vi "single-rev.vi"() -> ()   [LabVIEW 2020]
uses:
  rev_meas/Device_state.ctl
  GlobalDeviceNum1.vi
  support/Message Queue/Message Queue.lvlib
  support/User Event - Stop/User Event - Stop.lvlib
  setup/support/rev_setup.lvlib
  rev_meas/rev_meas.lvlib
  bas_meas/bas_meas.lvlib
panel:
  out "待处理删除数量":i32
  in  "校准":bool
  in  "EM设置":bool
  in  "HW设置":bool
  in  "退出":bool
  in  "开始":bool
  in  "选项卡控件":enum32{"当前结果", "记录结果", "分析结果"}(tab)
  out "当前混响频谱图":cluster{dbl[], "所有X坐标":dbl[]}(graph)
  in  "T1":bool
  in  "T2":bool
  in  "当前混响结果":i32(listbox)
  out "测量状态":string
  out "队列中元素数量":i32
  in  "deletelineT1":bool
  in  "clearlistT1":bool
  in  "deletelineT2":bool
  in  "clearlistT2":bool
  in  "T1结果":i32(listbox)
  in  "T2结果":i32(listbox)
  in  "All results":i32(listbox)
  in  "analysis":bool
  out "欢迎":string="欢迎使用"
  out "日期/时间字符串":string
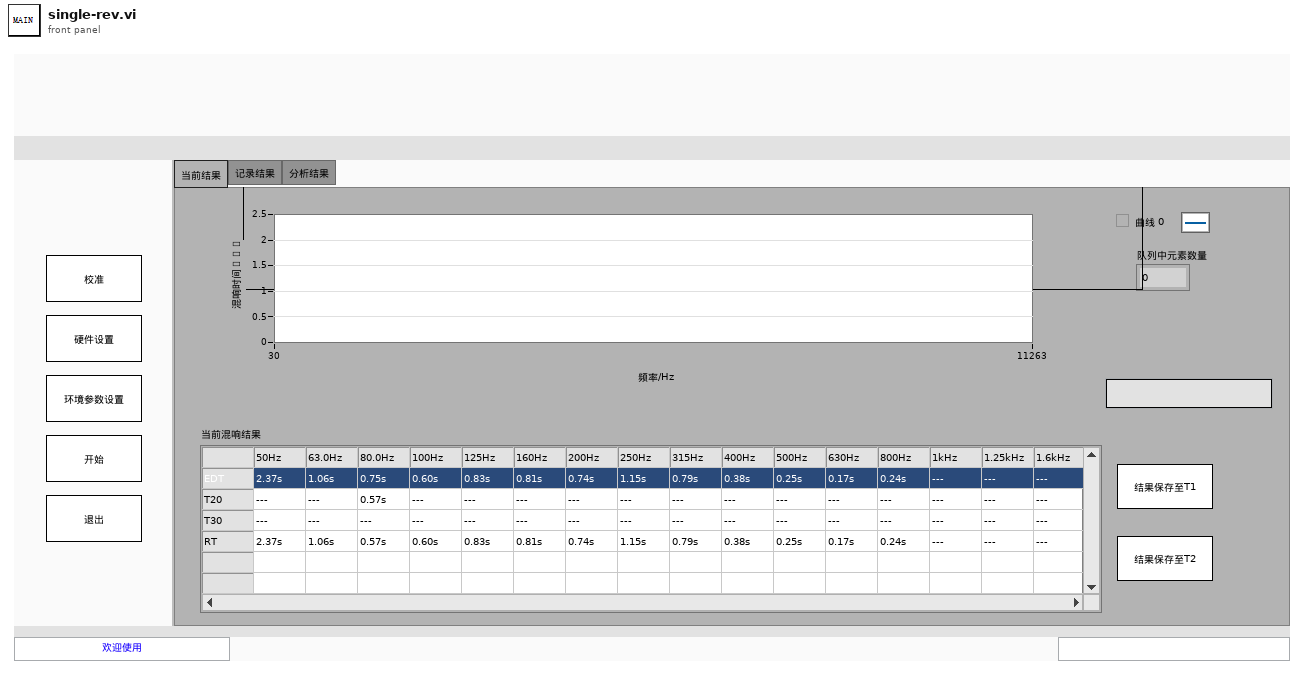
[diagram p1: front panel]
types:
  T1 = typedef "rev_meas.lvlib/Device_state.ctl" = enum16{"Idel", "testing", "stoped"}
  T2 = typedef "Message Queue.lvlib/All Message Queues.ctl" = cluster{"UI":refnum<queue>, "采集":refnum<queue>, "记录":refnum<queue>}
  T3 = cluster{"T1":dbl[], "T2":dbl[], "A1":dbl[], "A2":dbl[], "AT":dbl[], "Aobj":dbl[], "αs":dbl[]}
  T4 = cluster{"T1":string[], "T2":string[], "A1":string[], "A2":string[], "AT":string[], "Aobj":string[], "αs":string[]}
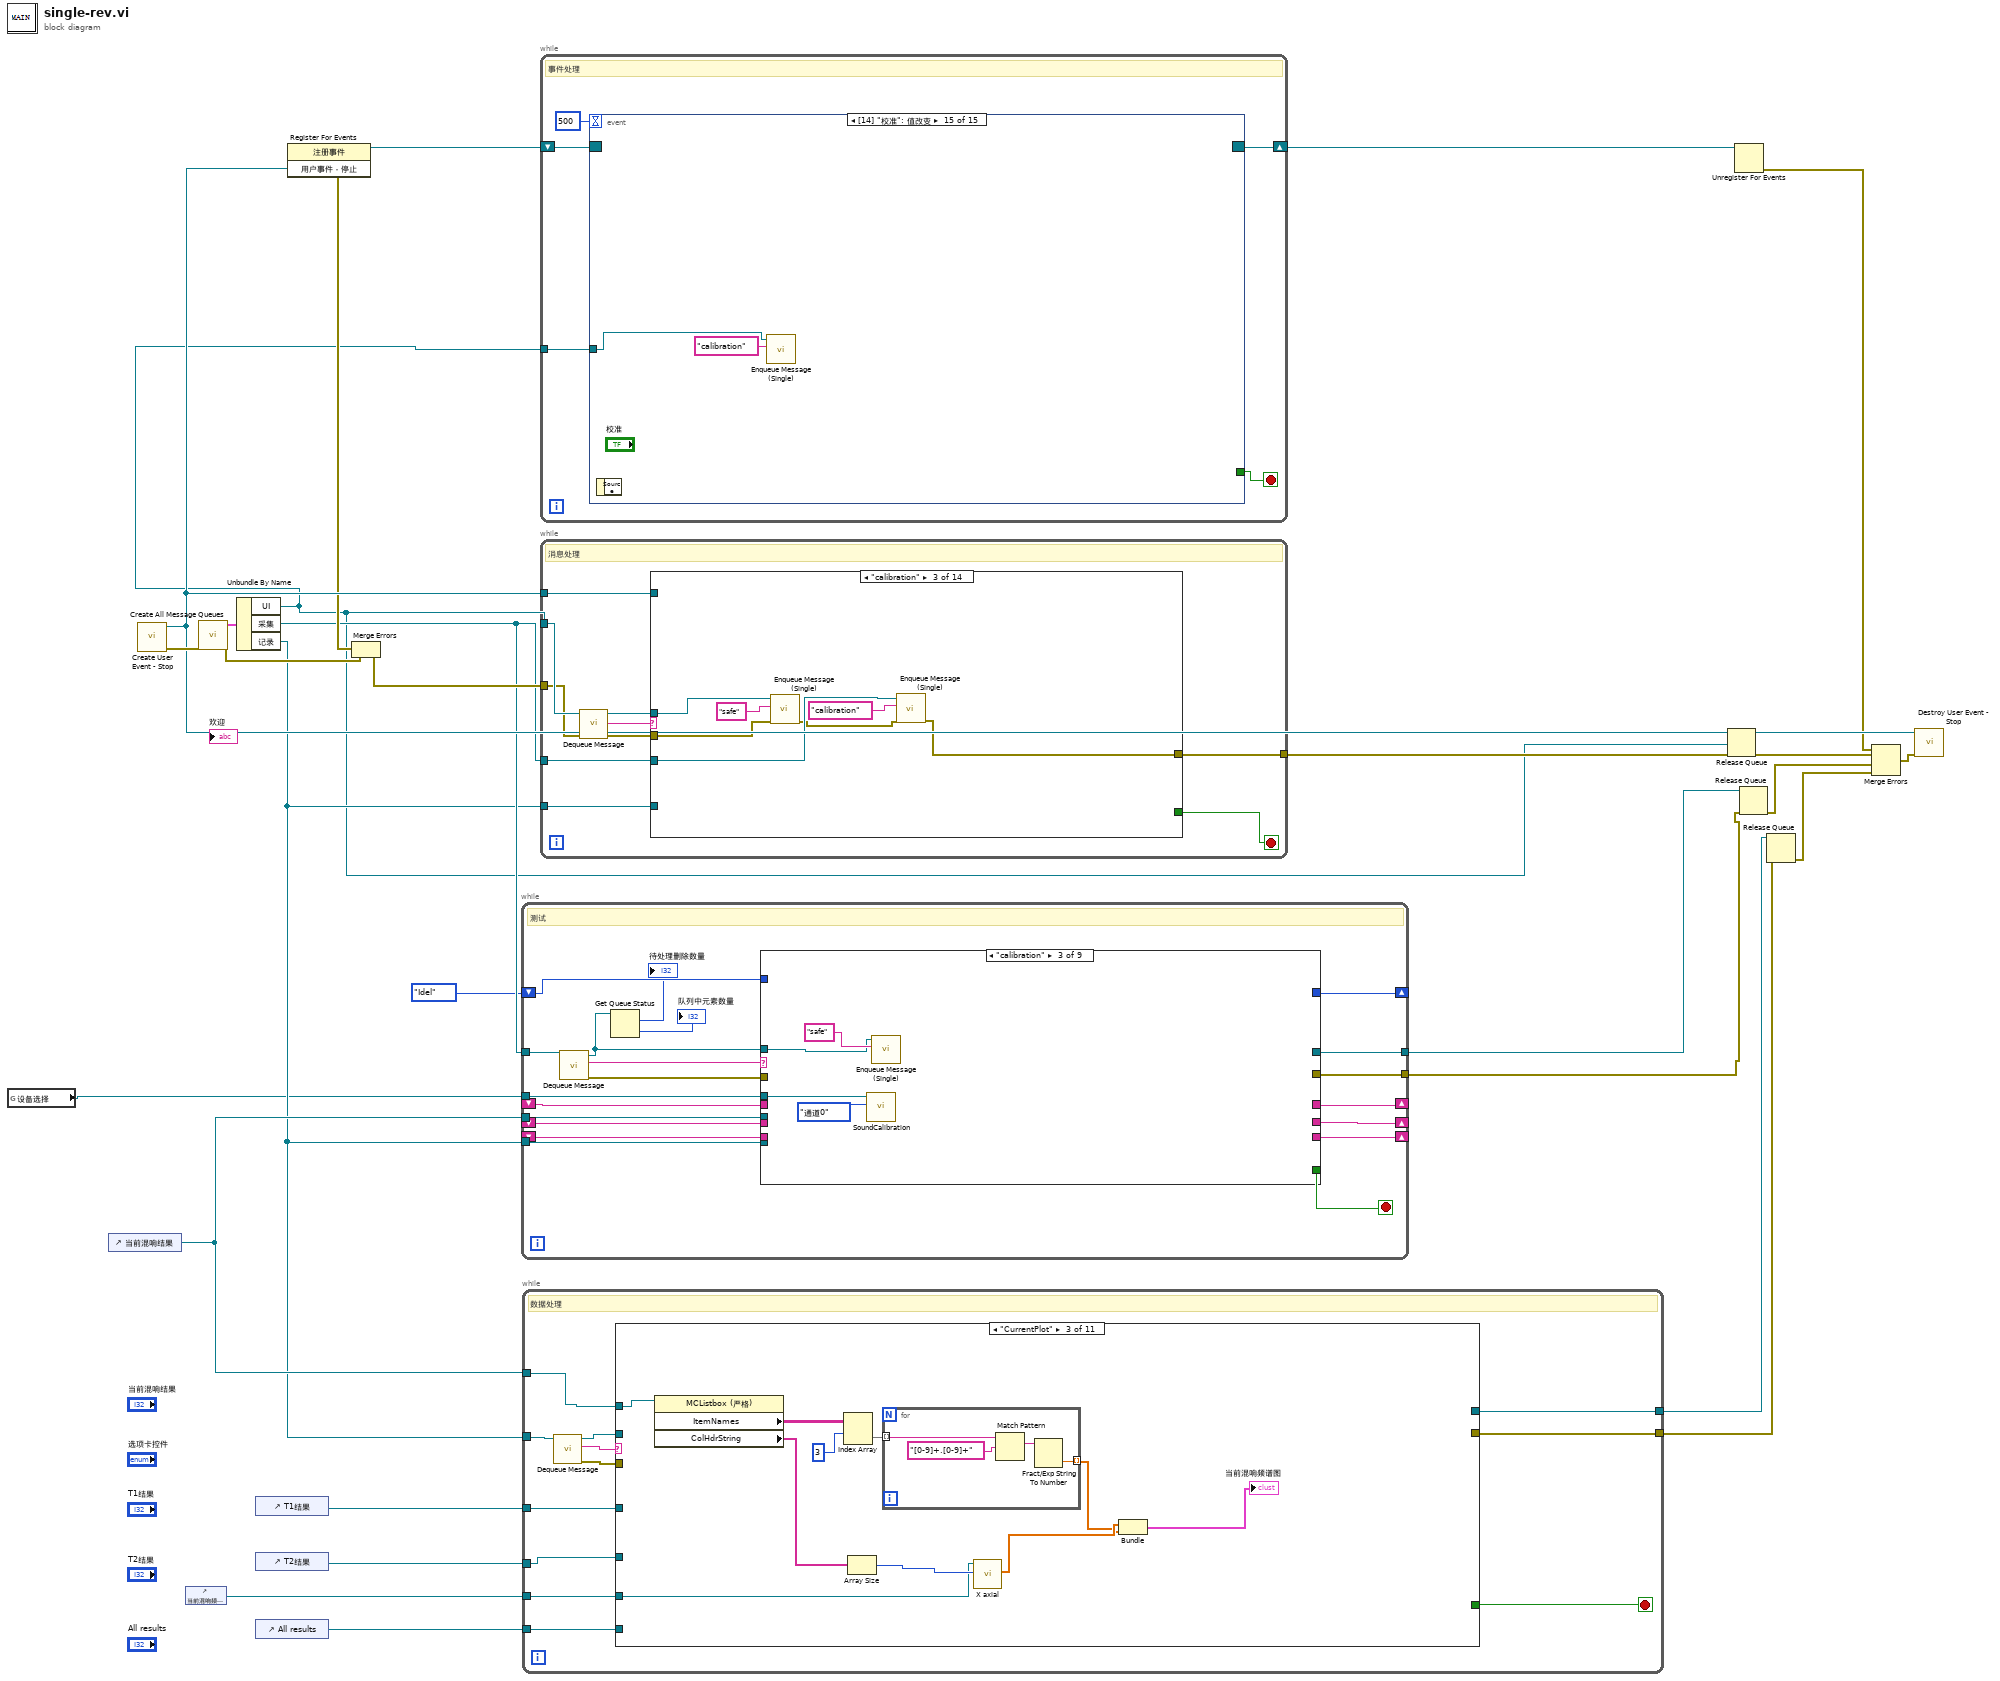
[diagram p0: block diagram]
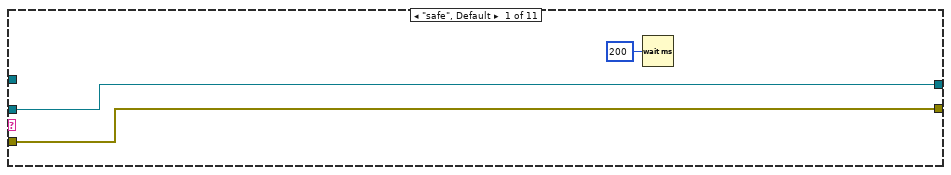
[diagram p2: hidden frame]
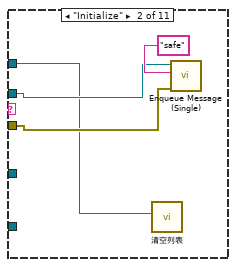
[diagram p3: hidden frame]
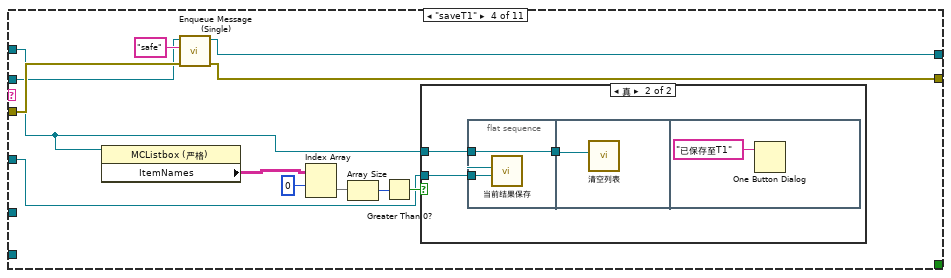
[diagram p4: hidden frame]
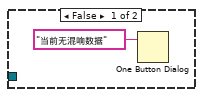
[diagram p5: hidden frame]
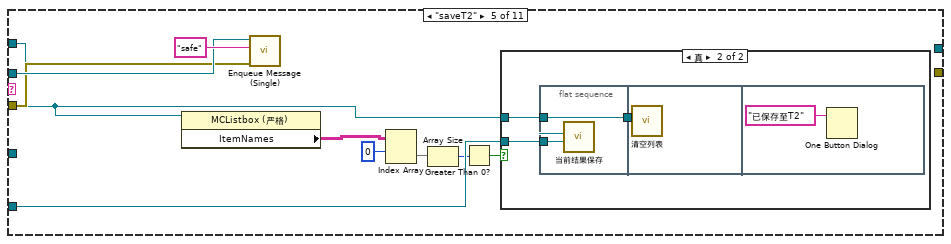
[diagram p6: hidden frame]
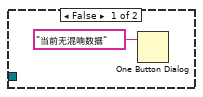
[diagram p7: hidden frame]
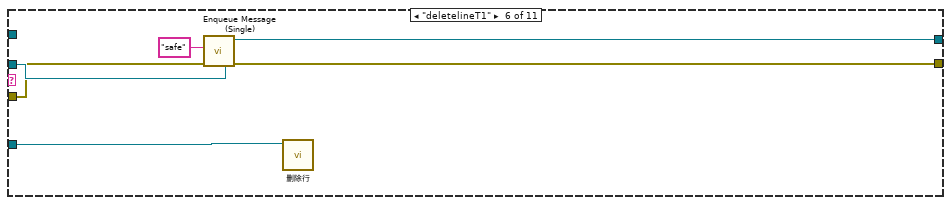
[diagram p8: hidden frame]
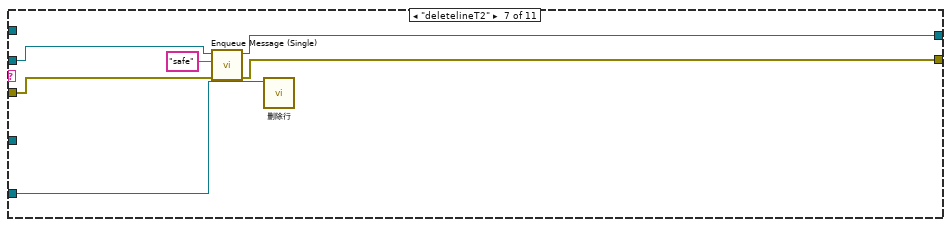
[diagram p9: hidden frame]
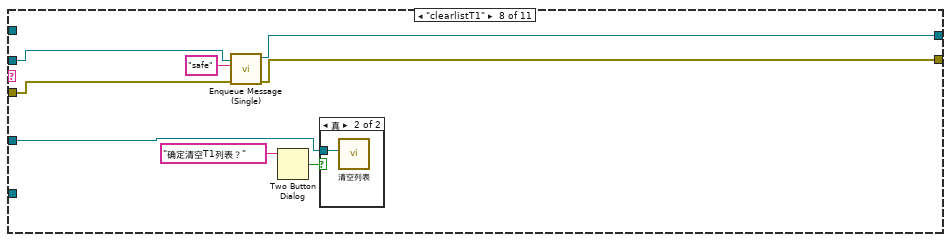
[diagram p10: hidden frame]
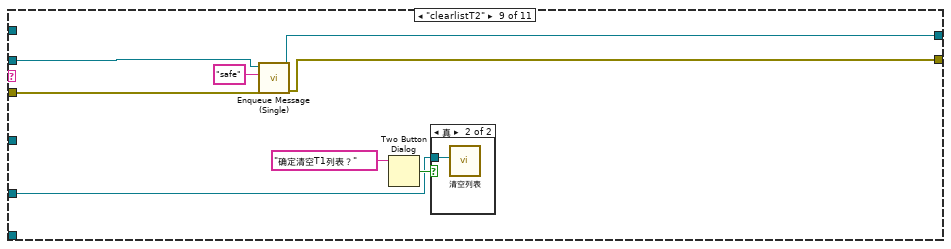
[diagram p12: hidden frame]
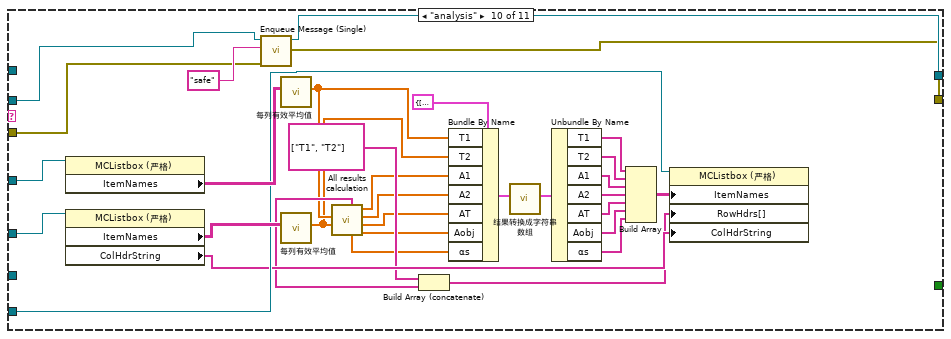
[diagram p14: hidden frame]
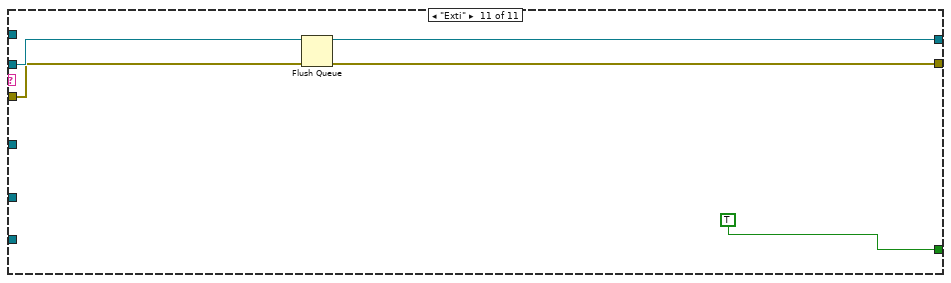
[diagram p15: hidden frame]
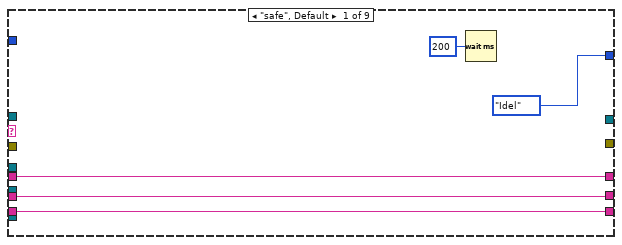
[diagram p16: hidden frame]
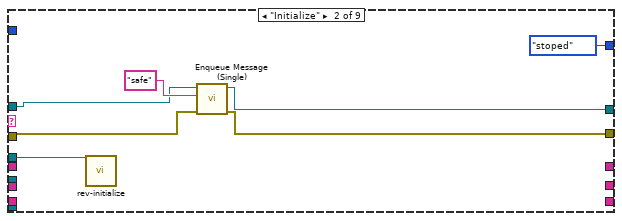
[diagram p17: hidden frame]
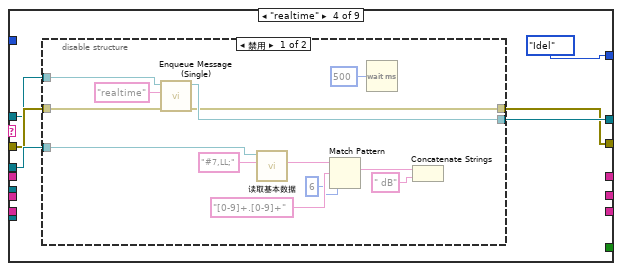
[diagram p18: hidden frame]
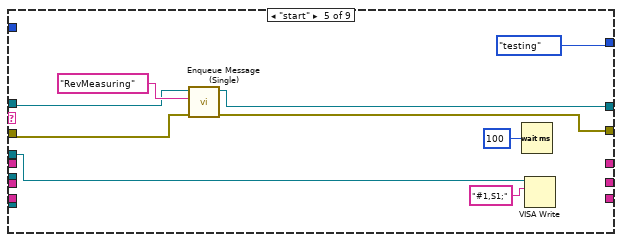
[diagram p20: hidden frame]
diagram:
  n1 = global read "GlobalDeviceNum1.vi" "设备选择"() -> (w4:refnum<visa-resource-name>)
  n2 = control-ref of="当前混响结果"() -> (w9:refnum<vi>)
  n3 = call "Create User Event - Stop.vi"() -> ("error out"=w26:cluster{"状态":bool, "代码":i32, "源":string}, "用户事件－停止"=w25:refnum<user-event>)  [unwired: 10 in]
  n4 = control-ref of="当前混响频谱图"() -> (w2:refnum<vi>)
  n5 = call "Create All Message Queues.vi"("error in (no error)"=w26) -> ("error out"=w23:cluster{"状态":bool, "代码":i32, "源":string}, "消息队列输出"=w28:T2)  [unwired: 9 in]
  n6 = Unbundle By Name(w28) -> ("UI"=w3:refnum<queue>, "采集"=w19:refnum<queue>, "记录"=w6:refnum<queue>)
  n7 = control-ref of="T1结果"() -> (w8:refnum<vi>)
  n8 = control-ref of="T2结果"() -> (w7:refnum<vi>)
  n9 = control-ref of="All results"() -> (w5:refnum<vi>)
  n10 = register-events(w25) -> (reference out=w27:refnum<event-registration>, error out=w22:errorcluster)  [unwired: 2 in]
  n11 = Merge Errors(w22, w23) -> (w21:errorcluster)
  n12 = while {
    tunnel: w4 -> [w46]
    tunnel: w9 -> [w43]
    tunnel: [w41] -> w11
    tunnel: w6 -> [w40]
    shift-right: [w39] -> _
    shift-left: _ -> [w36]
    shift-right: [w38] -> _
    shift-left: _ -> [w35]
    shift-right: [w37] -> _
    shift-left: _ -> [w34]
    shift-right: [w33] -> _
    shift-left: Device_state."Idel" ("枚举") -> [w32]
    tunnel: w19 -> [w48]
    tunnel: [w42] -> w15
    stop <- w44 stop-if-true
    # "测试"
    n13 = call "Dequeue Message.vi"("消息队列"=w48) -> ("error out"=w47:cluster{"状态":bool, "代码":i32, "源":string}, "消息"=w45:string, "消息队列副本"=w30:refnum<queue>)  [unwired: 7 in, 1 out]
    n14 = Get Queue Status(queue=w30) -> (# pending remove=→"待处理删除数量":i32, # elements in queue=→"队列中元素数量":i32)  [unwired: 2 in, 6 out]
    n15 = case shown="\"calibration\"" w45 {
      tunnel: w30 -> [_ w59 w61 w67 w88 w93 w133 w137 w145]
      tunnel: w47 -> [_ w58 _ w68 w87 w100 w132 w136 w143]
      tunnel: w46 -> [_ w55 w64 w69 w90 w102 _ w139 _]
      tunnel: [_ _ _ _ _ _ _ _ TRUE] -> w44
      tunnel: w43 -> [_ _ _ _ _ _ w121 _ _]
      tunnel: [_ w57 _ w66 w86 w95 w118 _ w144] -> w42
      tunnel: [_ w56 _ w65 w85 w94 w113 _ w142] -> w41
      tunnel: w40 -> [_ _ _ _ _ _ w119 _ _]
      tunnel: [w52 _ _ _ _ w99 _ _ _] -> w39
      tunnel: [w51 _ _ _ _ w98 _ _ _] -> w38
      tunnel: [w50 _ _ _ _ w97 _ _ _] -> w37
      tunnel: w36 -> [w52 _ _ _ _ _ w131 _ _]
      tunnel: w35 -> [w51 _ _ _ _ _ w130 _ _]
      tunnel: w34 -> [w50 _ _ _ _ _ w129 _ _]
      tunnel: [Device_state."Idel" ("枚举") Device_state."stoped" ("枚举") _ Device_state."Idel" ("枚举") Device_state."testing" ("枚举") Device_state."testing" ("枚举") Device_state."Idel" ("枚举") _ _] -> w33
      tunnel: w32 -> [_ _ _ _ _ _ _ _ _]
      frame "safe", Default {
        n16 = Wait (ms)(milliseconds to wait=u32 200 ("等待时间（毫秒）")) -> ()  [unwired: 1 out]
      }
      frame "Initialize" {
        n17 = call "rev-initialize.vi"("设备选择"=w55) -> ()  [unwired: 11 in]
        n18 = call "Enqueue Message (Single).vi"("error in (no error)"=w58, "消息"="safe", "消息队列"=w59) -> ("error out"=w56:cluster{"状态":bool, "代码":i32, "源":string}, "消息队列副本"=w57:refnum<queue>)  [unwired: 7 in]
      }
      frame "calibration" {
        n19 = call "SoundCalibration.vi"("通道选择"=enum16{"通道0", "通道1", "通道2", "通道3"}."通道0", "设备选择"=w64) -> ()  [unwired: 10 in]
        n20 = call "Enqueue Message (Single).vi"("消息"="safe", "消息队列"=w61) -> ()  [unwired: 8 in, 2 out]
      }
      frame "realtime" {
        n21 = disable-structure shown="禁用" {
          disable-tunnel: w69 -> [w83 _]
          disable-tunnel: w68 -> [w82 _]
          disable-tunnel: w67 -> [w81 _]
          disable-tunnel: [w80 _] -> w66
          disable-tunnel: [w79 _] -> w65
          frame Disabled {
            n22 = call "Enqueue Message (Single).vi"("error in (no error)"=w82, "消息"="realtime", "消息队列"=w81) -> ("error out"=w79:cluster{"状态":bool, "代码":i32, "源":string}, "消息队列副本"=w80:refnum<queue>)  [unwired: 7 in]
            n23 = call "读取基本数据.vi"("写入缓冲区"="#7,LL;", "设备选择"=w83) -> ("read buffer"=w77:string)  [unwired: 9 in]
            n24 = Match Pattern(string=w77, regular expression="[0-9]+.[0-9]+" ("正则表达式"), offset (0)=6 ("偏移量(0)")) -> (match substring=w78:string)  [unwired: 3 out]
            n25 = Wait (ms)(milliseconds to wait=u32 500 ("等待时间（毫秒）")) -> ()  [unwired: 1 out]
            n26 = Concatenate Strings(w78, " dB" ("字符串")) -> ()  [unwired: 1 out]
          }
          frame Enabled {
          }
        }
      }
      frame "start" {
        n27 = call "Enqueue Message (Single).vi"("error in (no error)"=w87, "消息"="RevMeasuring", "消息队列"=w88) -> ("error out"=w85:cluster{"状态":bool, "代码":i32, "源":string}, "消息队列副本"=w86:refnum<queue>)  [unwired: 7 in]
        n28 = Wait (ms)(milliseconds to wait=u32 100 ("等待时间（毫秒）")) -> ()  [unwired: 1 out]
        n29 = VISA Write(VISA resource name=w90, write buffer="#1,S1;" ("写入缓冲区")) -> ()  [unwired: 1 in, 3 out]
      }
      frame "RevMeasuring" {
        n30 = call "971A混响时间测量sub-单次读取.vi"("VISA资源名称"=w102) -> ("测量状态"=w101:string, "EDT结果"=w99:string, "T20结果"=w98:string, "T30结果"=w97:string)  [unwired: 10 in, 1 out]
        "测量状态" <- w101
        n31 = case shown="\"假\", 默认" w101 {
          tunnel: w100 -> [w106 _]
          tunnel: w93 -> [w107 w111]
          tunnel: [w104 w110] -> w95
          tunnel: [w105 w109] -> w94
          frame "假", Default {
            n32 = call "Enqueue Message (Single).vi"("优先消息？ (F)"=FALSE, "error in (no error)"=w106, "消息"="RevMeasuring", "消息队列"=w107) -> ("error out"=w105:cluster{"状态":bool, "代码":i32, "源":string}, "消息队列副本"=w104:refnum<queue>)  [unwired: 6 in]
          }
          frame "测量完成" {
            n33 = call "Enqueue Message (Single).vi"("消息"="RevProcessing", "消息队列"=w111) -> ("error out"=w109:cluster{"状态":bool, "代码":i32, "源":string}, "消息队列副本"=w110:refnum<queue>)  [unwired: 8 in]
          }
        }
      }
      frame "RevProcessing" {
        n34 = call "971A混响数据处理sub.vi"("EDT输入"=w131, "T20输入"=w130, "T30输入"=w129) -> ("频率输出"=w123:string[], "EDT输出"=w128:string[], "T20输出"=w127:string[], "T30输出"=w126:string[])  [unwired: 9 in]
        n35 = call "混响结果判断.vi"("T30数组"=w126, "T20数组"=w127, "EDT数组"=w128) -> ("RT result"=w125:string[])  [unwired: 8 in]
        n36 = call "Enqueue Message (Single).vi"("error in (no error)"=w132, "消息"="safe", "消息队列"=w133) -> ("error out"=w115:cluster{"状态":bool, "代码":i32, "源":string}, "消息队列副本"=w118:refnum<queue>)  [unwired: 7 in]
        n37 = Build Array(w128, w127, w126, w125) -> (w122:string[][])
        n38 = property class="MCListbox (严格)"(reference=w121, "ItemNames"=w122, "ColHdrString"=w123, "RowHdrs[]"=string[] ["EDT", "T20", "T30", "RT"]) -> (error out=w116:errorcluster)  [unwired: 1 in, 1 out]
        n39 = call "Enqueue Message (Single).vi"("error in (no error)"=w116, "消息"="CurrentPlot", "消息队列"=w119) -> ("error out"=w114:cluster{"状态":bool, "代码":i32, "源":string})  [unwired: 7 in, 1 out]
        n40 = Merge Errors(w115, w114) -> (w113:errorcluster)
      }
      frame "HWsetup" {
        n41 = flat-sequence {
          tunnel: w139 -> [w140]
          tunnel: [w140] -> w135
          tunnel: w135 -> [w141]
          frame #0 {
            n42 = call "HWsetup options.vi"("设备选择"=w140) -> ()  [unwired: 11 in]
          }
          frame #1 {
            n43 = VISA Clear(VISA resource name=w141) -> ()  [unwired: 1 in, 2 out]
          }
        }
        n44 = call "Enqueue Message (Single).vi"("error in (no error)"=w136, "消息"="safe", "消息队列"=w137) -> ()  [unwired: 7 in, 2 out]
      }
      frame "Exti" {
        n45 = Flush Queue(queue=w145, error in (no error)=w143) -> (queue out=w144:refnum<queue>, error out=w142:errorcluster)  [unwired: 1 out]
      }
    }
  }
  n46 = while {
    tunnel: w6 -> [w157]
    tunnel: w9 -> [w155]
    tunnel: [w152] -> w13
    tunnel: [w151] -> w10
    tunnel: w8 -> [w150]
    tunnel: w7 -> [w149]
    tunnel: w5 -> [w148]
    tunnel: w2 -> [w147]
    stop <- w156 stop-if-true
    # "数据处理"
    n47 = call "Dequeue Message.vi"("消息队列"=w157) -> ("error out"=w153:cluster{"状态":bool, "代码":i32, "源":string}, "消息"=w158:string, "消息队列副本"=w154:refnum<queue>)  [unwired: 7 in, 1 out]
    n48 = case shown="\"CurrentPlot\"" w158 {
      tunnel: [_ _ _ _ _ _ _ _ _ _ TRUE] -> w156
      tunnel: w155 -> [_ w162 w166 w180 w205 _ _ _ _ _ _]
      tunnel: w154 -> [w160 w164 _ w187 w208 w222 w228 w234 w242 w278 w283]
      tunnel: w153 -> [w159 w163 _ w190 w207 w221 w227 w233 w243 w277 w281]
      tunnel: [w160 _ _ w189 _ w220 w226 w236 w245 w276 w282] -> w152
      tunnel: [w159 _ _ w188 _ w219 w225 w235 w244 w275 w280] -> w151
      tunnel: w150 -> [_ _ _ w181 _ w218 _ w230 _ w274 _]
      tunnel: w149 -> [_ _ _ _ w206 _ w224 _ w239 w273 _]
      tunnel: w148 -> [_ _ _ _ _ _ _ _ _ w270 _]
      tunnel: w147 -> [_ _ w169 _ _ _ _ _ _ _ _]
      frame "safe", Default {
        n49 = Wait (ms)(milliseconds to wait=u32 200 ("等待时间（毫秒）")) -> ()  [unwired: 1 out]
      }
      frame "Initialize" {
        n50 = call "清空列表.vi"("列表"=w162) -> ()  [unwired: 11 in]
        n51 = call "Enqueue Message (Single).vi"("error in (no error)"=w163, "消息"="safe", "消息队列"=w164) -> ()  [unwired: 7 in, 2 out]
      }
      frame "CurrentPlot" {
        n52 = property class="MCListbox (严格)"(reference=w166) -> ("ItemNames"=w175:string[][], "ColHdrString"=w172:string[])  [unwired: 1 in, 2 out]
        n53 = Index Array(array=w175, index (row)=3 ("索引 (行)")) -> (element=w173:string[])  [unwired: 1 in]
        n54 = Array Size(array=w172) -> (size(s)=w171:i32)
        n55 = for {
          tunnel: w173 -> [w179] mode=indexing
          tunnel: [w176] -> w167 mode=indexing
          n56 = Match Pattern(string=w179, regular expression="[0-9]+.[0-9]+" ("正则表达式")) -> (match substring=w177:string)  [unwired: 1 in, 3 out]
          n57 = Fract/Exp String To Number(string=w177) -> (number=w176:dbl)  [unwired: 3 in, 1 out]
        }
        n58 = call "X axial.vi"("频率配置"=w171, "当前混响频谱图 2"=w169) -> ("所有X坐标"=w168:dbl[])  [unwired: 9 in]
        n59 = Bundle("所有X坐标"=w168, w167) -> (→"当前混响频谱图":cluster{"所有X坐标":dbl[], dbl[]})  [unwired: 1 in]
      }
      frame "saveT1" {
        n60 = property class="MCListbox (严格)"(reference=w180) -> ("ItemNames"=w185:string[][])  [unwired: 1 in, 2 out]
        n61 = call "Enqueue Message (Single).vi"("error in (no error)"=w190, "消息"="safe", "消息队列"=w187) -> ("error out"=w188:cluster{"状态":bool, "代码":i32, "源":string}, "消息队列副本"=w189:refnum<queue>)  [unwired: 7 in]
        n62 = Index Array(array=w185, index (row)=0 ("索引 (行)")) -> (element=w183:string[])  [unwired: 1 in]
        n63 = Array Size(array=w183) -> (size(s)=w186:i32)
        n64 = Greater Than 0?(x=w186) -> (x > 0?=w182:bool)
        n65 = case shown="真" w182 {
          tunnel: w181 -> [_ w195]
          tunnel: w180 -> [_ w194]
          frame False {
            n66 = One Button Dialog(message="当前无混响数据" ("消息")) -> ()  [unwired: 1 in, 1 out]
          }
          frame True {
            n67 = flat-sequence {
              tunnel: w195 -> [w197]
              tunnel: w194 -> [w196]
              tunnel: [w196] -> w193
              tunnel: w193 -> [w198]
              frame #0 {
                n68 = call "当前结果保存.vi"("列表2"=w197, "列表1"=w196) -> ()  [unwired: 10 in]
              }
              frame #1 {
                n69 = call "清空列表.vi"("列表"=w198) -> ()  [unwired: 11 in]
              }
              frame #2 {
                n70 = One Button Dialog(message="已保存至T1" ("消息")) -> ()  [unwired: 1 in, 1 out]
              }
            }
          }
        }
      }
      frame "saveT2" {
        n71 = property class="MCListbox (严格)"(reference=w205) -> ("ItemNames"=w203:string[][])  [unwired: 1 in, 2 out]
        n72 = call "Enqueue Message (Single).vi"("error in (no error)"=w207, "消息"="safe", "消息队列"=w208) -> ()  [unwired: 7 in, 2 out]
        n73 = Index Array(array=w203, index (row)=0 ("索引 (行)")) -> (element=w201:string[])  [unwired: 1 in]
        n74 = Array Size(array=w201) -> (size(s)=w204:i32)
        n75 = Greater Than 0?(x=w204) -> (x > 0?=w200:bool)
        n76 = case shown="真" w200 {
          tunnel: w206 -> [_ w213]
          tunnel: w205 -> [_ w212]
          frame False {
            n77 = One Button Dialog(message="当前无混响数据" ("消息")) -> ()  [unwired: 1 in, 1 out]
          }
          frame True {
            n78 = flat-sequence {
              tunnel: w213 -> [w215]
              tunnel: w212 -> [w214]
              tunnel: [w214] -> w211
              tunnel: w211 -> [w216]
              frame #0 {
                n79 = call "当前结果保存.vi"("列表2"=w215, "列表1"=w214) -> ()  [unwired: 10 in]
              }
              frame #1 {
                n80 = call "清空列表.vi"("列表"=w216) -> ()  [unwired: 11 in]
              }
              frame #2 {
                n81 = One Button Dialog(message="已保存至T2" ("消息")) -> ()  [unwired: 1 in, 1 out]
              }
            }
          }
        }
      }
      frame "deletelineT1" {
        n82 = call "Enqueue Message (Single).vi"("error in (no error)"=w221, "消息"="safe", "消息队列"=w222) -> ("error out"=w219:cluster{"状态":bool, "代码":i32, "源":string}, "消息队列副本"=w220:refnum<queue>)  [unwired: 7 in]
        n83 = call "删除行.vi"("列表"=w218) -> ()  [unwired: 11 in]
      }
      frame "deletelineT2" {
        n84 = call "Enqueue Message (Single).vi"("error in (no error)"=w227, "消息"="safe", "消息队列"=w228) -> ("error out"=w225:cluster{"状态":bool, "代码":i32, "源":string}, "消息队列副本"=w226:refnum<queue>)  [unwired: 7 in]
        n85 = call "删除行.vi"("列表"=w224) -> ()  [unwired: 11 in]
      }
      frame "clearlistT1" {
        n86 = call "Enqueue Message (Single).vi"("error in (no error)"=w233, "消息"="safe", "消息队列"=w234) -> ("error out"=w235:cluster{"状态":bool, "代码":i32, "源":string}, "消息队列副本"=w236:refnum<queue>)  [unwired: 7 in]
        n87 = Two Button Dialog(message="确定清空T1列表？" ("消息")) -> (T button?=w231:bool)  [unwired: 2 in]
        n88 = case shown="真" w231 {
          tunnel: w230 -> [_ w238]
          frame False {
          }
          frame True {
            n89 = call "清空列表.vi"("列表"=w238) -> ()  [unwired: 11 in]
          }
        }
      }
      frame "clearlistT2" {
        n90 = call "Enqueue Message (Single).vi"("error in (no error)"=w243, "消息"="safe", "消息队列"=w242) -> ("error out"=w244:cluster{"状态":bool, "代码":i32, "源":string}, "消息队列副本"=w245:refnum<queue>)  [unwired: 7 in]
        n91 = Two Button Dialog(message="确定清空T1列表？" ("消息")) -> (T button?=w240:bool)  [unwired: 2 in]
        n92 = case shown="真" w240 {
          tunnel: w239 -> [_ w247]
          frame False {
          }
          frame True {
            n93 = call "清空列表.vi"("列表"=w247) -> ()  [unwired: 11 in]
          }
        }
      }
      frame "analysis" {
        n94 = property class="MCListbox (严格)"(reference=w274) -> ("ItemNames"=w272:string[][])  [unwired: 1 in, 2 out]
        n95 = property class="MCListbox (严格)"(reference=w273) -> ("ItemNames"=w271:string[][], "ColHdrString"=w269:string[])  [unwired: 1 in, 2 out]
        n96 = call "Enqueue Message (Single).vi"("error in (no error)"=w277, "消息"="safe", "消息队列"=w278) -> ("error out"=w275:cluster{"状态":bool, "代码":i32, "源":string}, "消息队列副本"=w276:refnum<queue>)  [unwired: 7 in]
        n97 = call "每列有效平均值.vi"("测试数组"=w272) -> ("平均混响时间"=w265:dbl[])  [unwired: 10 in]
        n98 = call "每列有效平均值.vi"("测试数组"=w271) -> ("平均混响时间"=w264:dbl[])  [unwired: 10 in]
        n99 = call "All results calculation.vi"("平均混响时间T2"=w264, "平均混响时间T1"=w265) -> ("分立吸声体吸声量Aobj"=w260:dbl[], "试件吸声量AT"=w261:dbl[], "混响室吸声量A2"=w262:dbl[], "混响室吸声量A1"=w263:dbl[], "吸声系数αs"=w259:dbl[], "rowhead"=w267:string[])  [unwired: 4 in]
        n100 = Build Array (concatenate)(string[] ["T1", "T2"], w267) -> (w248:string[])
        n101 = Bundle By Name(cluster=T3 {"T1"=[], "T2"=[], "A1"=[], "A2"=[], "AT"=[], "Aobj"=[], "αs"=[]} ("结果数据数组簇"), "T1"=w265, "T2"=w264, "A1"=w263, "A2"=w262, "AT"=w261, "Aobj"=w260, "αs"=w259) -> (w258:T3)
        n102 = call "结果转换成字符串数组.vi"("结果数据数组簇"=w258) -> ("结果字符串数组簇"=w257:T4)  [unwired: 10 in]
        n103 = Unbundle By Name(w257) -> ("T1"=w256:string[], "T2"=w255:string[], "A1"=w254:string[], "A2"=w253:string[], "AT"=w252:string[], "Aobj"=w251:string[], "αs"=w250:string[])
        n104 = Build Array(w256, w255, w254, w253, w252, w251, w250) -> (w249:string[][])
        n105 = property class="MCListbox (严格)"(reference=w270, "ItemNames"=w249, "RowHdrs[]"=w248, "ColHdrString"=w269) -> ()  [unwired: 1 in, 2 out]
      }
      frame "Exti" {
        n106 = Flush Queue(queue=w283, error in (no error)=w281) -> (queue out=w282:refnum<queue>, error out=w280:errorcluster)  [unwired: 1 out]
      }
    }
  }
  n107 = while {
    tunnel: w3 -> [w288]
    shift-right: [w286] -> w24
    shift-left: w27 -> [w287]
    stop <- w289 stop-if-true
    # "事件处理"
    n108 = event shown="[14] \"校准\": 值改变" {
      selector: w287 -> [_ _ _ _ _ _ _ _ _ _ _ _ _ _ _]
      dyn-events: [_ _ _ _ _ _ _ _ _ _ _ _ _ _ _] -> w286
      timeout: 500 -> [_ _ _ _ _ _ _ _ _ _ _ _ _ _ _]
      tunnel: [_ w294 _ _ _ _ TRUE _ _ _ _ _ _ _ _] -> w289
      tunnel: w288 -> [_ w291 w296 w297 w300 w302 _ w305 w307 w309 w311 w313 w315 w317 w319]
      event Timeout {
        n109 = event-data() -> ()  [unwired: 1 in, 3 out]
        n110 = Format Date/Time String() -> (date/time string=→"日期/时间字符串":string)  [unwired: 3 in]
      }
      event Panel Close? {
        w294 = TRUE ("放弃？")
        n111 = event-data() -> ()  [unwired: 1 in, 4 out]
        n112 = call "Enqueue Message (Single).vi"("优先消息？ (F)"=TRUE, "消息"="Exti", "消息队列"=w291) -> ()  [unwired: 7 in, 2 out]
        n113 = event-data("Discard?"=w294) -> ()  [unwired: 1 in, 1 out]
      }
      event "HW设置": Value Change {
        n114 = event-data() -> ()  [unwired: 1 in, 1 out]
        n115 = call "Enqueue Message (Single).vi"("消息"="HWsetup", "消息队列"=w296) -> ()  [unwired: 8 in, 2 out]
      }
      event "EM设置": Value Change {
        n116 = event-data() -> ()  [unwired: 1 in, 1 out]
        n117 = call "Enqueue Message (Single).vi"("消息"="EMsetup", "消息队列"=w297) -> ()  [unwired: 8 in, 2 out]
      }
      event "开始": Value Change {
        n118 = event-data() -> ()  [unwired: 1 in, 1 out]
        n119 = call "Enqueue Message (Single).vi"("消息"="start", "消息队列"=w300) -> ()  [unwired: 8 in, 2 out]
      }
      event "退出": Value Change {
        n120 = event-data() -> ()  [unwired: 1 in, 1 out]
        n121 = call "Enqueue Message (Single).vi"("优先消息？ (F)"=TRUE, "消息"="Exti", "消息队列"=w302) -> ()  [unwired: 7 in, 2 out]
      }
      event User Event {
        n122 = event-data() -> ()  [unwired: 1 in, 1 out]
      }
      event "T1": Value Change {
        n123 = event-data() -> ()  [unwired: 1 in, 1 out]
        n124 = call "Enqueue Message (Single).vi"("消息"="saveT1", "消息队列"=w305) -> ()  [unwired: 8 in, 2 out]
      }
      event "T2": Value Change {
        n125 = event-data() -> ()  [unwired: 1 in, 1 out]
        n126 = call "Enqueue Message (Single).vi"("消息"="saveT2", "消息队列"=w307) -> ()  [unwired: 8 in, 2 out]
      }
      event "deletelineT1": Value Change {
        n127 = event-data() -> ()  [unwired: 1 in, 1 out]
        n128 = call "Enqueue Message (Single).vi"("消息"="deletelineT1", "消息队列"=w309) -> ()  [unwired: 8 in, 2 out]
      }
      event "deletelineT2": Value Change {
        n129 = event-data() -> ()  [unwired: 1 in, 1 out]
        n130 = call "Enqueue Message (Single).vi"("消息"="deletelineT2", "消息队列"=w311) -> ()  [unwired: 8 in, 2 out]
      }
      event "clearlistT1": Value Change {
        n131 = event-data() -> ()  [unwired: 1 in, 1 out]
        n132 = call "Enqueue Message (Single).vi"("消息"="clearlistT1", "消息队列"=w313) -> ()  [unwired: 8 in, 2 out]
      }
      event "clearlistT2": Value Change {
        n133 = event-data() -> ()  [unwired: 1 in, 1 out]
        n134 = call "Enqueue Message (Single).vi"("消息"="clearlistT2", "消息队列"=w315) -> ()  [unwired: 8 in, 2 out]
      }
      event "analysis": Value Change {
        n135 = event-data() -> ()  [unwired: 1 in, 1 out]
        n136 = call "Enqueue Message (Single).vi"("消息"="analysis", "消息队列"=w317) -> ()  [unwired: 8 in, 2 out]
      }
      event "校准": Value Change {
        n137 = event-data() -> ()  [unwired: 1 in, 1 out]
        n138 = call "Enqueue Message (Single).vi"("消息"="calibration", "消息队列"=w319) -> ()  [unwired: 8 in, 2 out]
      }
    }
  }
  n139 = while {
    tunnel: w3 -> [w330]
    tunnel: w25 -> [w328]
    tunnel: w21 -> [w326]
    tunnel: [w325] -> w20
    tunnel: w19 -> [w322]
    tunnel: w6 -> [w321]
    stop <- w327 stop-if-true
    # "消息处理"
    n140 = call "Dequeue Message.vi"("error in (no error)"=w326, "消息队列"=w330) -> ("error out"=w323:cluster{"状态":bool, "代码":i32, "源":string}, "消息"=w329:string, "消息队列副本"=w324:refnum<queue>)  [unwired: 6 in, 1 out]
    n141 = case shown="\"calibration\"" w329 {
      tunnel: w328 -> [_ _ _ _ _ _ _ _ _ _ _ _ _ w413]
      tunnel: [_ _ _ _ _ _ _ _ _ _ _ _ _ TRUE] -> w327
      tunnel: [w331 w333 w337 w344 _ w355 w358 _ w371 _ w384 w394 w398 w411] -> w325
      tunnel: w324 -> [_ w335 w342 w347 _ w356 w361 w367 w374 w380 w386 w392 w399 w405]
      tunnel: w323 -> [w331 w334 w341 w345 _ w353 w359 w365 w372 w379 w385 w393 w400 _]
      tunnel: w322 -> [_ _ w339 w346 _ w354 _ _ _ _ _ _ _ w410]
      tunnel: w321 -> [_ _ _ _ _ _ w360 w366 w373 w378 w387 w391 w401 w408]
      frame "safe", Default {
        n142 = Wait (ms)(milliseconds to wait=u32 20 ("等待时间（毫秒）")) -> ()  [unwired: 1 out]
      }
      frame "Initialize" {
        n143 = call "Enqueue Message (Single).vi"("error in (no error)"=w334, "消息"="safe", "消息队列"=w335) -> ("error out"=w333:cluster{"状态":bool, "代码":i32, "源":string})  [unwired: 7 in, 1 out]
      }
      frame "calibration" {
        n144 = call "Enqueue Message (Single).vi"("error in (no error)"=w341, "消息"="safe", "消息队列"=w342) -> ("error out"=w338:cluster{"状态":bool, "代码":i32, "源":string})  [unwired: 7 in, 1 out]
        n145 = call "Enqueue Message (Single).vi"("error in (no error)"=w338, "消息"="calibration", "消息队列"=w339) -> ("error out"=w337:cluster{"状态":bool, "代码":i32, "源":string})  [unwired: 7 in, 1 out]
      }
      frame "HWsetup" {
        n146 = call "Enqueue Message (Single).vi"("error in (no error)"=w345, "消息"="HWsetup", "消息队列"=w346) -> ("error out"=w349:cluster{"状态":bool, "代码":i32, "源":string})  [unwired: 7 in, 1 out]
        n147 = call "Enqueue Message (Single).vi"("error in (no error)"=w349, "消息"="safe", "消息队列"=w347) -> ("error out"=w344:cluster{"状态":bool, "代码":i32, "源":string})  [unwired: 7 in, 1 out]
      }
      frame "EMsetup" {
        n148 = call "EMsetup options.vi"() -> ()  [unwired: 12 in]
      }
      frame "start" {
        n149 = call "Enqueue Message (Single).vi"("error in (no error)"=w353, "消息"="start", "消息队列"=w354) -> ("error out"=w352:cluster{"状态":bool, "代码":i32, "源":string})  [unwired: 7 in, 1 out]
        n150 = call "Enqueue Message (Single).vi"("error in (no error)"=w352, "消息"="safe", "消息队列"=w356) -> ("error out"=w355:cluster{"状态":bool, "代码":i32, "源":string})  [unwired: 7 in, 1 out]
      }
      frame "saveT1" {
        n151 = call "Enqueue Message (Single).vi"("error in (no error)"=w359, "消息"="saveT1", "消息队列"=w360) -> ("error out"=w363:cluster{"状态":bool, "代码":i32, "源":string})  [unwired: 7 in, 1 out]
        n152 = call "Enqueue Message (Single).vi"("error in (no error)"=w363, "消息"="safe", "消息队列"=w361) -> ("error out"=w358:cluster{"状态":bool, "代码":i32, "源":string})  [unwired: 7 in, 1 out]
      }
      frame "saveT2" {
        n153 = call "Enqueue Message (Single).vi"("error in (no error)"=w365, "消息"="saveT2", "消息队列"=w366) -> ("error out"=w370:cluster{"状态":bool, "代码":i32, "源":string})  [unwired: 7 in, 1 out]
        n154 = call "Enqueue Message (Single).vi"("error in (no error)"=w370, "消息"="safe", "消息队列"=w367) -> ()  [unwired: 7 in, 2 out]
      }
      frame "deletelineT1" {
        n155 = call "Enqueue Message (Single).vi"("error in (no error)"=w372, "消息"="deletelineT1", "消息队列"=w373) -> ("error out"=w377:cluster{"状态":bool, "代码":i32, "源":string})  [unwired: 7 in, 1 out]
        n156 = call "Enqueue Message (Single).vi"("error in (no error)"=w377, "消息"="safe", "消息队列"=w374) -> ("error out"=w371:cluster{"状态":bool, "代码":i32, "源":string})  [unwired: 7 in, 1 out]
      }
      frame "deletelineT2" {
        n157 = call "Enqueue Message (Single).vi"("error in (no error)"=w379, "消息"="deletelineT2", "消息队列"=w378) -> ("error out"=w383:cluster{"状态":bool, "代码":i32, "源":string})  [unwired: 7 in, 1 out]
        n158 = call "Enqueue Message (Single).vi"("error in (no error)"=w383, "消息"="safe", "消息队列"=w380) -> ()  [unwired: 7 in, 2 out]
      }
      frame "clearlistT1" {
        n159 = call "Enqueue Message (Single).vi"("error in (no error)"=w385, "消息"="clearlistT1", "消息队列"=w387) -> ("error out"=w390:cluster{"状态":bool, "代码":i32, "源":string})  [unwired: 7 in, 1 out]
        n160 = call "Enqueue Message (Single).vi"("error in (no error)"=w390, "消息"="safe", "消息队列"=w386) -> ("error out"=w384:cluster{"状态":bool, "代码":i32, "源":string})  [unwired: 7 in, 1 out]
      }
      frame "clearlistT2" {
        n161 = call "Enqueue Message (Single).vi"("error in (no error)"=w393, "消息"="clearlistT2", "消息队列"=w391) -> ("error out"=w397:cluster{"状态":bool, "代码":i32, "源":string})  [unwired: 7 in, 1 out]
        n162 = call "Enqueue Message (Single).vi"("error in (no error)"=w397, "消息"="safe", "消息队列"=w392) -> ("error out"=w394:cluster{"状态":bool, "代码":i32, "源":string})  [unwired: 7 in, 1 out]
      }
      frame "analysis" {
        n163 = call "Enqueue Message (Single).vi"("error in (no error)"=w400, "消息"="analysis", "消息队列"=w401) -> ("error out"=w404:cluster{"状态":bool, "代码":i32, "源":string})  [unwired: 7 in, 1 out]
        n164 = call "Enqueue Message (Single).vi"("error in (no error)"=w404, "消息"="safe", "消息队列"=w399) -> ("error out"=w398:cluster{"状态":bool, "代码":i32, "源":string})  [unwired: 7 in, 1 out]
      }
      frame "Exti" {
        w406 = "Exti" ("消息")
        n165 = call "Enqueue Message (Single).vi"("优先消息？ (F)"=TRUE, "消息"=w406, "消息队列"=w410) -> ()  [unwired: 7 in, 2 out]
        n166 = call "Enqueue Message (Single).vi"("优先消息？ (F)"=TRUE, "消息"=w406, "消息队列"=w408) -> ()  [unwired: 7 in, 2 out]
        n167 = call "Fire User Event - Stop.vi"("用户事件－停止"=w413) -> ("error out"=w411:cluster{"状态":bool, "代码":i32, "源":string})  [unwired: 10 in]
        n168 = Flush Queue(queue=w405) -> ()  [unwired: 1 in, 3 out]
      }
    }
  }
  n169 = Release Queue(queue=w3, error in (no error)=w20) -> (error out=w16:errorcluster)  [unwired: 1 in, 2 out]
  n170 = Unregister For Events(event registration refnum=w24) -> (error out=w17:errorcluster)  [unwired: 1 in]
  n171 = Release Queue(queue=w15, error in (no error)=w11) -> (error out=w14:errorcluster)  [unwired: 1 in, 2 out]
  n172 = Release Queue(queue=w13, error in (no error)=w10) -> (error out=w12:errorcluster)  [unwired: 1 in, 2 out]
  n173 = Merge Errors(w17, w16, w14, w12) -> (w18:errorcluster)
  n174 = call "Destroy User Event - Stop.vi"("error in (no error)"=w18, "用户事件－停止"=w25) -> ()  [unwired: 9 in, 1 out]
